vi "All Read RF BIN without indicator and warmup.vi"() -> (3 "All Toolkit Times":T1 {"Accelerator CUDA Time" format="%#_gs"; "Accelerator TRT Time" format="%#_gs"; "Culab Time" format="%#_gs"; "G2CPU Time" format="%#_gs"; "LabVIEW Time" format="%#_gs"})   [LabVIEW 2020]
doc: "Execute GEMM Process for different size on different Toolkits (Accelerator/Culab/CUDA/LabVIEW/G2CPU) and LabVIEW(CPU)."
uses:
  Source/_Controls/acc_execution_provider_enum.ctl
  <vilib>/Natan Biesmans/G2CPU GPU and CPU HPC Toolkit/ArrayFire Driver/TypeDefs/backend.ctl
  <vilib>/Natan Biesmans/G2CPU GPU and CPU HPC Toolkit/ArrayFire Driver/AF.lvlib
panel:
  out "G2CPU Time":dbl format="%#_gs"
  out "LabVIEW Time":dbl format="%#_gs"
  out "Accelerator CUDA Time":dbl format="%#_gs"
  out "Culab Time":dbl format="%#_gs"
  out "Accelerator TRT Time":dbl format="%#_gs"
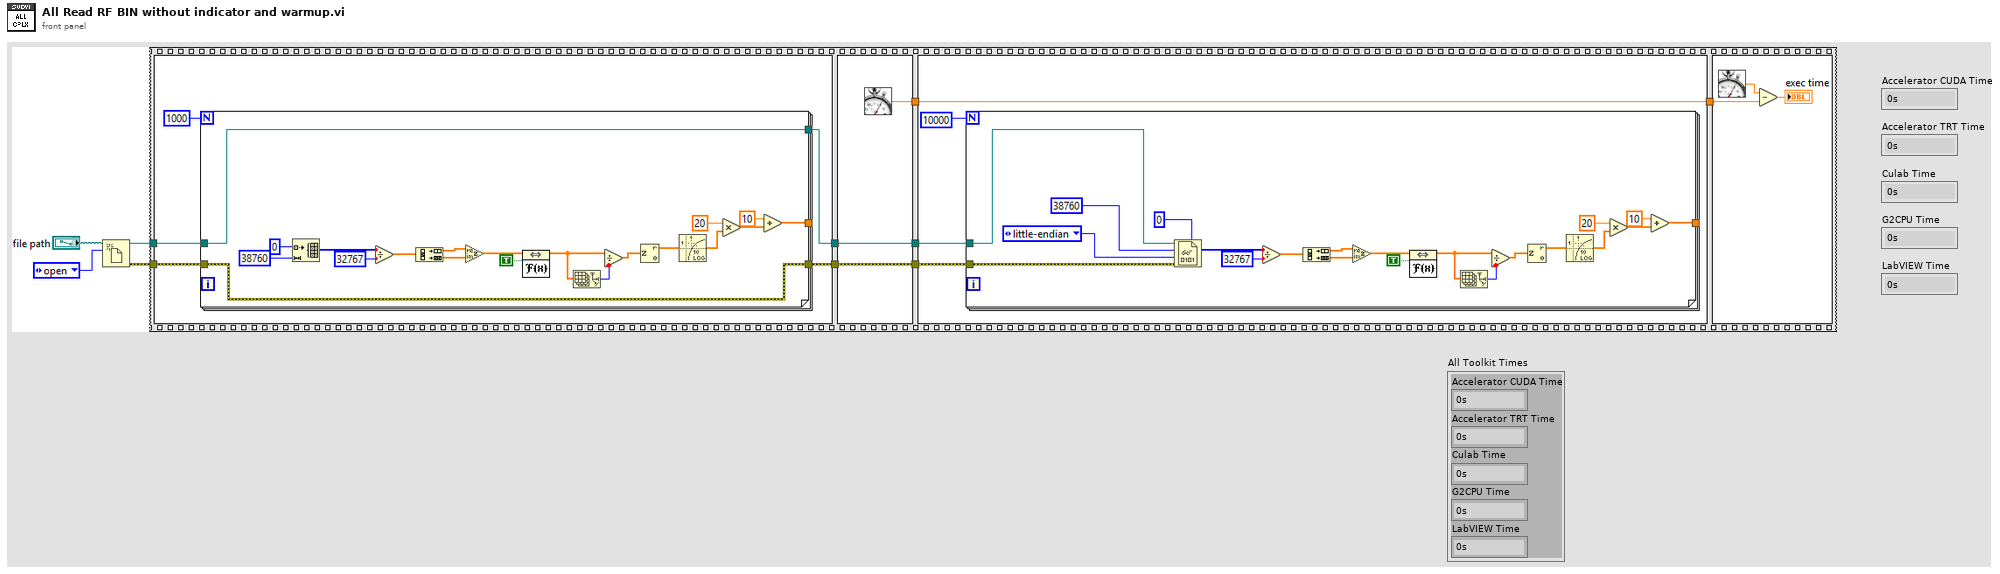
[diagram p1: front panel]
types:
  T1 = cluster{"Accelerator CUDA Time":dbl, "Accelerator TRT Time":dbl, "Culab Time":dbl, "G2CPU Time":dbl, "LabVIEW Time":dbl}
  T2 = cluster{"intra_op_num_threads":i32, "inter_op_num_threads":i32, "execution_mode":enum16{"ORT_SEQUENTIAL", "ORT_PARALLEL"}, "deterministic_compute":bool, "graph_optimization_level":u16, "optimized_model_file_path":path, "profiling output dir":path}
  T3 = typedef "acc_execution_provider_enum.ctl" = enum16{"CPU", "CUDA", "TensorRT"}
  T4 = typedef "AF.lvlib/backend.ctl" = u32
  T5 = cluster{"exec time":dbl, "exec time":dbl, "exec time":dbl, "time":dbl, "exec time":dbl}
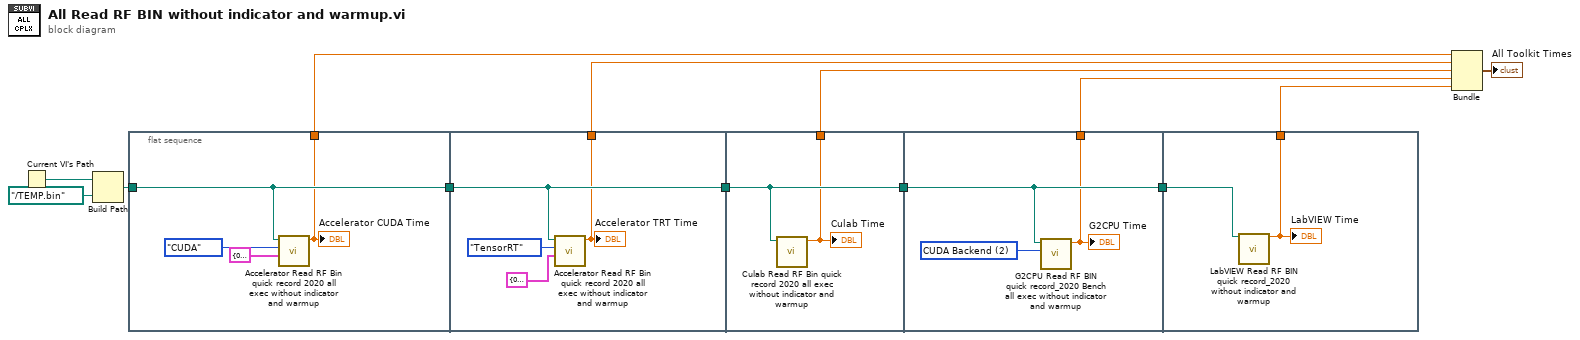
[diagram p0: block diagram]
diagram:
  n1 = Current VI's Path() -> (path=w13:path)
  n2 = Build Path(base path=w13, name or relative path=path "../TEMP.bin") -> (appended path=w11:path)
  n3 = flat-sequence {
    tunnel: w11 -> [w15]
    tunnel: [w15] -> w10
    tunnel: [w14] -> w6
    tunnel: w10 -> [w19]
    tunnel: [w19] -> w9
    tunnel: [w18] -> w5
    tunnel: w9 -> [w23]
    tunnel: [w23] -> w8
    tunnel: [w22] -> w4
    tunnel: w8 -> [w25]
    tunnel: [w25] -> w7
    tunnel: [w24] -> w3
    tunnel: w7 -> [w28]
    tunnel: [w27] -> w2
    frame #0 {
      n4 = call "Accelerator Read RF Bin quick record 2020 all exec without indicator and warmup.vi"("Sessions Parameters"=T2 {"intra_op_num_threads"=0, "inter_op_num_threads"=0, "execution_mode"=enum."ORT_SEQUENTIAL", "deterministic_compute"=FALSE, "graph_optimization_level"=1, "optimized_model_file_path"=path "", "profiling output dir"=path ""}, "Execution Device"=acc_execution_provider_enum."CUDA", "file path"=w15) -> ("exec time"=w14:dbl)  [unwired: 8 in]
      "Accelerator CUDA Time" <- w14
    }
    frame #1 {
      n5 = call "Accelerator Read RF Bin quick record 2020 all exec without indicator and warmup.vi"("Sessions Parameters"=T2 {"intra_op_num_threads"=0, "inter_op_num_threads"=0, "execution_mode"=enum."ORT_SEQUENTIAL", "deterministic_compute"=FALSE, "graph_optimization_level"=1, "optimized_model_file_path"=path "", "profiling output dir"=path ""}, "Execution Device"=acc_execution_provider_enum."TensorRT", "file path"=w19) -> ("exec time"=w18:dbl)  [unwired: 8 in]
      "Accelerator TRT Time" <- w18
    }
    frame #2 {
      n6 = call "Culab Read RF Bin quick record 2020 all exec without indicator and warmup.vi"("file path"=w23) -> ("exec time"=w22:dbl)  [unwired: 10 in]
      "Culab Time" <- w22
    }
    frame #3 {
      w26 = T4 2 items=["Default Backend"=0, "CPU Backend"=1, "CUDA Backend"=2, "OPENCL Backend"=4, "Intel OneAPI Backend"=8] ("Backend")
      n7 = call "G2CPU Read RF BIN quick record_2020 Bench all exec without indicator and warmup.vi"("Backend"=w26, "file path"=w25) -> ("time"=w24:dbl)  [unwired: 9 in]
      "G2CPU Time" <- w24
    }
    frame #4 {
      n8 = call "LabVIEW Read RF BIN quick record_2020 without indicator and warmup.vi"("file path"=w28) -> ("exec time"=w27:dbl)  [unwired: 14 in]
      "LabVIEW Time" <- w27
    }
  }
  n9 = Bundle("exec time"=w6, "exec time"=w5, "exec time"=w4, "time"=w3, "exec time"=w2) -> (→"All Toolkit Times":T5)  [unwired: 1 in]
